vi "Configure Serial Bus (SPI - Trigger).vi"(0 "VISA resource name":refnum<visa-resource-name>, 1 "MISO Data Pattern (XXXXXXXX)":string="XXXXXXXX", 2 "MOSI Data Pattern (XXXXXXXX)":string="XXXXXXXX", 3 "Data Pattern (XXXXXXXX)":string="XXXXXXXX", 5 "Serial Bus Name (1: Serial Bus 1)":i32(ring)=1 items=["Serial Bus 1"=1, "Serial Bus 2"=2], 7 "MISO Data Length (8 bits)":i32=8, 9 "Trigger Type (0: MOSI)":i32(ring) items=["MOSI", "MISO", "DATA"], 11 "error in (no error)":errorcluster, 12 "MOSI Data Length (8 bits)":i32=8, 13 "Data Length (8 bits)":i32=8) -> (4 "VISA resource name out":refnum<visa-resource-name>, 15 "error out":errorcluster)   [LabVIEW 2017, in "Agilent 2000 3000 X-Series.lvlib"]
doc: "Configures the trigger settings of SPI bus."
uses:
  Agilent 2000 3000 X-Series.lvlib
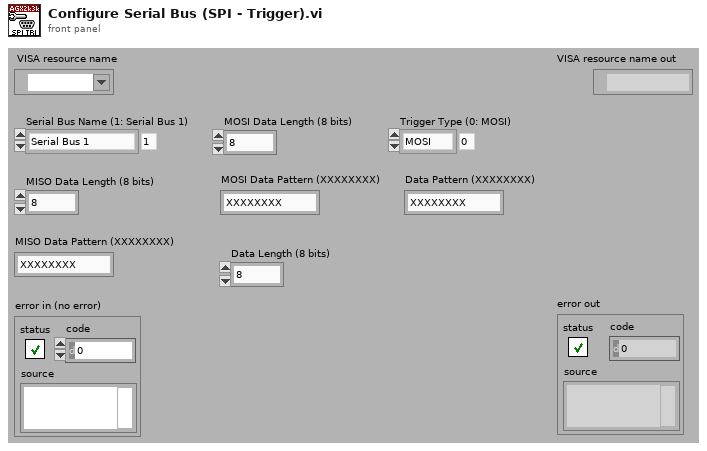
[diagram p1: front panel]
types:
  T1 = typedef "Agilent 2000 3000 X-Series.lvlib/Extended User Data.ctl" = cluster{"X-Series Mode":u16, "Acquisition Type (0: Normal)":i32}
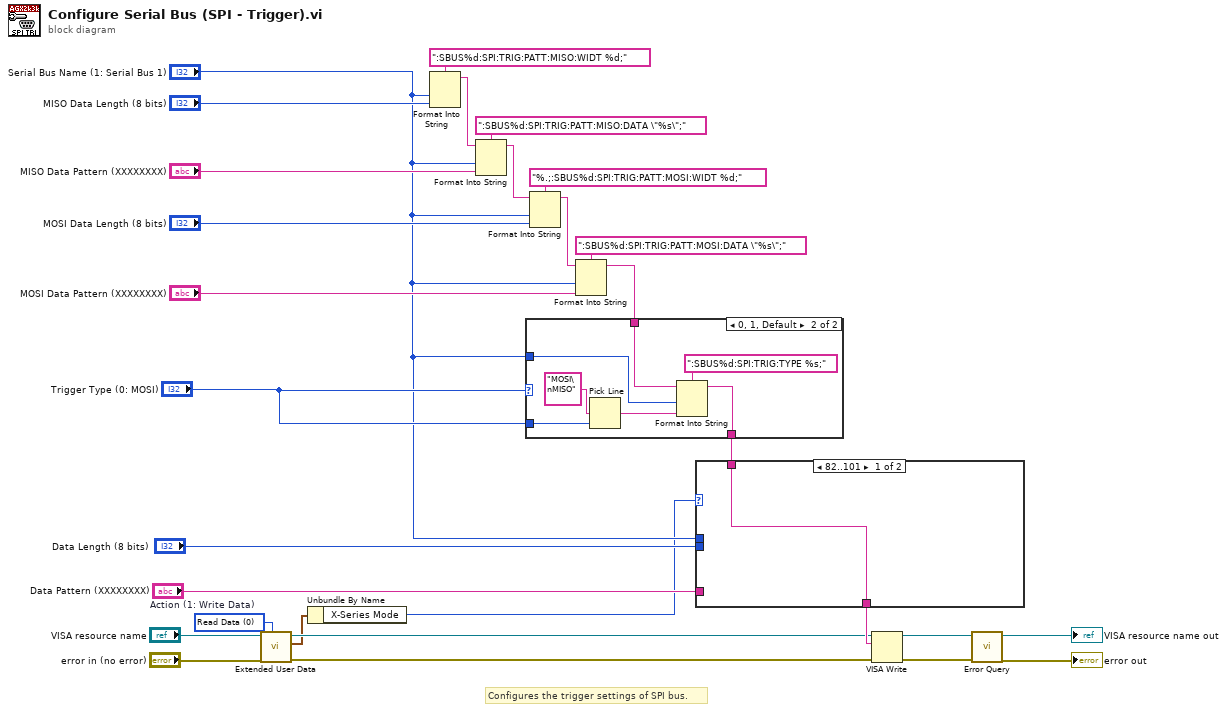
[diagram p0: block diagram]
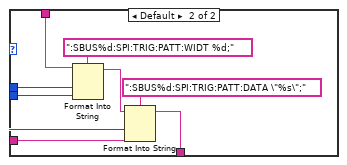
[diagram p2: hidden frame]
diagram:
  w2 = 0 items=["Read Data", "Write Data", "Clear Data", "Clear ALL Data"]  # Action (1: Write Data)
  # "Configures the trigger settings of SPI bus."
  n1 = call "Extended User Data.vi"("Action (1: Write Data)"=w2, "error in (no error)"="error in (no error)", "VISA resource name in"="VISA resource name") -> ("error out"=w4:errorcluster, "User Data Out"=w3:T1, "VISA resource name out"=w5:refnum<visa-resource-name>)  [unwired: 6 in]
  n2 = Unbundle By Name(w3) -> ("X-Series Mode"=w1:u16)
  n3 = Format Into String(format string=":SBUS%d:SPI:TRIG:PATT:MISO:WIDT %d;", "Serial Bus Name (1: Serial Bus 1)", "MISO Data Length (8 bits)") -> (resulting string=w17:string)  [unwired: 2 in, 1 out]
  n4 = Format Into String(format string=":SBUS%d:SPI:TRIG:PATT:MISO:DATA \"%s\";", initial string=w17, "Serial Bus Name (1: Serial Bus 1)", "MISO Data Pattern (XXXXXXXX)") -> (resulting string=w16:string)  [unwired: 1 in, 1 out]
  n5 = Format Into String(format string="%.;:SBUS%d:SPI:TRIG:PATT:MOSI:WIDT %d;", initial string=w16, "Serial Bus Name (1: Serial Bus 1)", "MOSI Data Length (8 bits)") -> (resulting string=w15:string)  [unwired: 1 in, 1 out]
  n6 = Format Into String(format string=":SBUS%d:SPI:TRIG:PATT:MOSI:DATA \"%s\";", initial string=w15, "Serial Bus Name (1: Serial Bus 1)", "MOSI Data Pattern (XXXXXXXX)") -> (resulting string=w13:string)  [unwired: 1 in, 1 out]
  n7 = case shown="0, 1, Default" "Trigger Type (0: MOSI)" {
    tunnel: "Trigger Type (0: MOSI)" -> [_ w37]
    tunnel: [w30 w31] -> w10
    tunnel: "Serial Bus Name (1: Serial Bus 1)" -> [_ w32]
    tunnel: w13 -> [w30 w34]
    frame 2 {
    }
    frame 0, 1, Default {
      n8 = Pick Line(multi-line string="MOSI\nMISO", line index=w37) -> (output string=w35:string)  [unwired: 1 out]
      n9 = Format Into String(format string=":SBUS%d:SPI:TRIG:TYPE %s;", initial string=w34, w32, w35) -> (resulting string=w31:string)  [unwired: 1 in, 1 out]
    }
  }
  n10 = case shown="82..101" w1 {
    tunnel: "Data Length (8 bits)" -> [_ w46]
    tunnel: "Data Pattern (XXXXXXXX)" -> [_ w45]
    tunnel: w10 -> [w38 w44]
    tunnel: "Serial Bus Name (1: Serial Bus 1)" -> [_ w41]
    tunnel: [w38 w39] -> w8
    frame 82..101 {
    }
    frame Default {
      n11 = Format Into String(format string=":SBUS%d:SPI:TRIG:PATT:WIDT %d;", initial string=w44, w41, w46) -> (resulting string=w42:string)  [unwired: 1 in, 1 out]
      n12 = Format Into String(format string=":SBUS%d:SPI:TRIG:PATT:DATA \"%s\";", initial string=w42, w41, w45) -> (resulting string=w39:string)  [unwired: 1 in, 1 out]
    }
  }
  n13 = VISA Write(VISA resource name=w5, write buffer=w8, error in (no error)=w4) -> (VISA resource name out=w21:refnum<visa-resource-name>, error out=w20:errorcluster)  [unwired: 1 out]
  n14 = call "Error Query.vi"("error in (no error)"=w20, "VISA resource name"=w21) -> ("error out"=→"error out":errorcluster, "VISA resource name out"=→"VISA resource name out":refnum<visa-resource-name>)  [unwired: 8 out]
